vi "Invalid profile name--error.vi"() -> (0 "error out":errorcluster)   [LabVIEW 2025]
doc: "Indicates that the provided profile name is invalid (Empty string)"
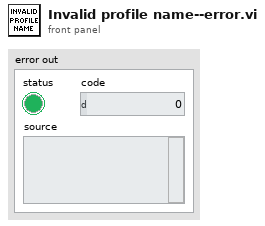
[diagram p1: front panel]
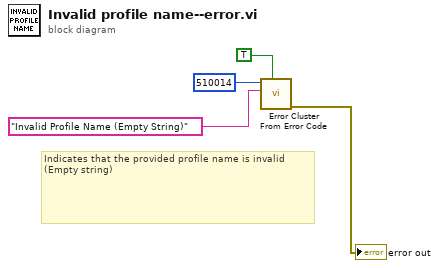
[diagram p0: block diagram]
diagram:
  # "Indicates that the provided profile name is invalid (Empty string)"
  n1 = call <vilib>:"Error Cluster From Error Code.vi"("show call chain? (False)"=TRUE, "error message (\"\")"="Invalid Profile Name (Empty String)" ("error message (\"\")"), "error code (0)"=510014) -> ("error out"=→"error out":errorcluster)  [unwired: 6 in]
